vi "to string.vi"(8 "error in":errorcluster, 11 "Scan Engine configuration in":refnum<class "Scan Engine configuration.lvclass">) -> (0 "error out":errorcluster, 1 "data":string, 2 "version":string, 3 "Scan Engine configuration out":refnum<class "Scan Engine configuration.lvclass">)   [LabVIEW 2013, in "Scan Engine configuration.lvclass"]
doc: "Provides an interface for saving a module configuration to a file or other serialized data source. It is recommended that all children of this class store data in two sets--data required for its own initialization, and any data required for parent initialization--and that each implementation uses the <b>Call Parent Method</b> primitive to serialize parent information."
uses:
  Scan Engine configuration.lvclass
  <vilib>/NI/Tag Bus Module Framework/module configuration/TBM module configuration.lvclass
  Scan Engine configuration.lvclass/Scan Engine configuration.ctl
  <vilib>/NI/Configuration Framework/serializable configuration/NISE_CEF_serializable configuration.lvclass
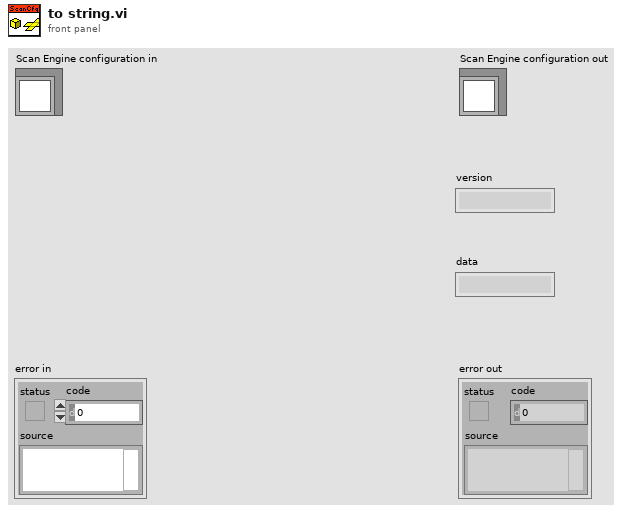
[diagram p1: front panel]
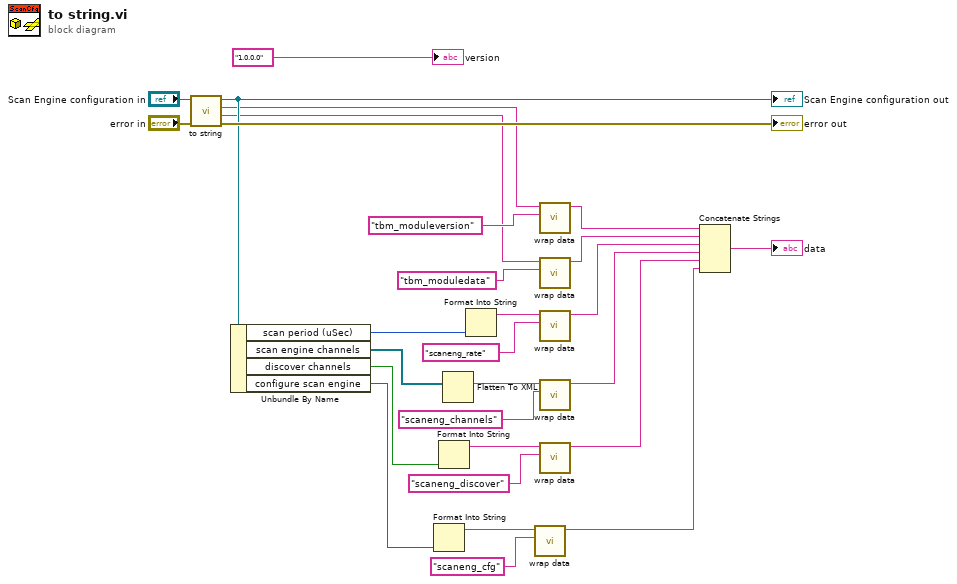
[diagram p0: block diagram]
diagram:
  n1 = call-parent "to string.vi"("error in"="error in", "module configuration in"="Scan Engine configuration in") -> ("error out"=→"error out":errorcluster, "data"=w16:string, "version"=w17:string, "module configuration out"=w18:refnum<class "Scan Engine configuration.lvclass">)  [unwired: 6 in]
  "Scan Engine configuration out" <- w18
  n2 = Unbundle By Name(w18) -> ("scan period (uSec)"=w14:u32, "scan engine channels"=w15:refnum<class "TBM channel.lvclass">[], "discover channels"=w9:bool, "configure scan engine"=w3:bool)
  n3 = Format Into String(w3) -> (resulting string=w4:string)  [unwired: 3 in, 1 out]
  n4 = Format Into String(w9) -> (resulting string=w8:string)  [unwired: 3 in, 1 out]
  n5 = Flatten To XML(anything=w15) -> (xml string=w21:string)
  n6 = Format Into String(w14) -> (resulting string=w13:string)  [unwired: 3 in, 1 out]
  n7 = call <vilib>:"wrap data.vi"("identifier"="scaneng_cfg" ("additional identifier"), "data to wrap"=w4) -> ("wrapped data"=w2:string)  [unwired: 9 in]
  n8 = call <vilib>:"wrap data.vi"("identifier"="tbm_moduleversion" ("additional identifier"), "data to wrap"=w17) -> ("wrapped data"=w23:string)  [unwired: 9 in]
  n9 = call <vilib>:"wrap data.vi"("identifier"="tbm_moduledata" ("additional identifier"), "data to wrap"=w16) -> ("wrapped data"=w22:string)  [unwired: 9 in]
  n10 = call <vilib>:"wrap data.vi"("identifier"="scaneng_rate" ("additional identifier"), "data to wrap"=w13) -> ("wrapped data"=w11:string)  [unwired: 9 in]
  n11 = call <vilib>:"wrap data.vi"("identifier"="scaneng_channels" ("additional identifier"), "data to wrap"=w21) -> ("wrapped data"=w20:string)  [unwired: 9 in]
  n12 = call <vilib>:"wrap data.vi"("identifier"="scaneng_discover" ("additional identifier"), "data to wrap"=w8) -> ("wrapped data"=w6:string)  [unwired: 9 in]
  n13 = Concatenate Strings(w23, w22, w11, w20, w6, w2) -> (→"data":string)
  "version" <- "1.0.0.0" ("current version")
